vi "aft_xmpl_Reference Sine Wave Generation.vi"(9 "Amplitude":dbl=1.0, 10 "order":dbl=1.0, 11 "Speed":dbl) -> (3 "Reference":dbl)   [LabVIEW 2019]
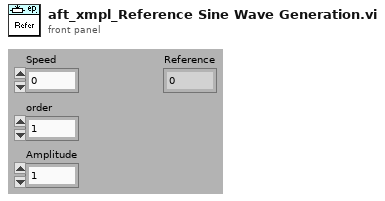
[diagram p1: front panel]
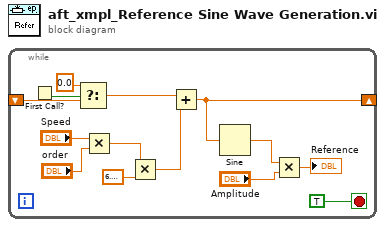
[diagram p0: block diagram]
diagram:
  n1 = while {
    shift-right: [w9] -> _
    shift-left: _ -> [w6]
    stop <- TRUE stop-if-true
    n2 = First Call?() -> (First Call?: T/F=w5:bool)
    n3 = Select(t=0.0, s=w5, f=w6) -> (s? t:f=w7:dbl)
    n4 = Multiply(x="Speed", y="order") -> (x*y=w10:dbl)
    n5 = Multiply(x=w10, y=6.283185307179586) -> (x*y=w13:dbl)
    n6 = Add(x=w7, y=w13) -> (x+y=w9:dbl)
    n7 = Sine(x=w9) -> (sin(x)=w3:dbl)
    n8 = Multiply(x=w3, y="Amplitude") -> (x*y=→"Reference":dbl)
  }
